vi "INIT TEMP.vi"(8 "error in (no error)":errorcluster, 9 "element":T2 {"Output's Control Loop (1:1)" items=["1"=1, "2"=2]; "Data Source (0:Kelvin)" items=["Kelvin", "Celsius", "Sensor Units"]; "Input (0:A)" items=["A", "B", "C", "D", "D2", "D3", "D4", "D5"]; "Configure Control Parameters (0: Configure)" items=["Configure", "Don't Configure"]; "Serial Configuration"."Flow Control" items=["None", "XON/XOFF", "RTS/CTS", "XON/XOFF & RTS/CTS", "DTR/DSR", "XON/XOFF & DTR/DSR"]; "Serial Configuration"."Stop Bits" items=["1.0"=10, "1.5"=15, "2.0"=20]; "Serial Configuration"."Data Bits" items=["7"=7, "8"=8]; "Serial Configuration"."Parity" items=["None", "Odd", "Even", "Mark", "Space"]; "Serial Configuration"."Baud Rate" items=["300"=300, "600"=600, "1200"=1200, "2400"=2400, "4800"=4800, "9600"=9600, "19200"=19200, "38400"=38400, "57600"=57600]; "Target Temp (K)" format="%.5f"; "Input (0:None)" items=["None", "A", "B", "C", "D", "D2", "D3", "D4", "D5"]; "Mode (0:Off)" items=["Off", "Closed Loop PID", "Zone", "Open Loop"]; "Heater Out Display (1:Current)" items=["Current"=1, "Power"=2]; "Max Current (0:User Specified)" items=["User Specified", "0.707 A", "1.0 A", "1.141 A", "2.0 A"]; "Heater Resistance (1:25 Ohms)" items=["25 Ohms"=1, "50 Ohms"=2]; "Max User Current (2.000)" format="%.3f"; "Gain (P) (50.0)" format="%.1f"; "Reset (I) (20.0)" format="%.1f"; "Rate (D) (0.0 %)" format="%.1f"; "Manual Output (0.00 %)" format="%.2f"; "Range (0:Off)" items=["Off", "Range 1 (On)", "Range 2", "Range 3", "Range 4", "Range 5"]}, 10 "Field and Temp Range":T1={"VISA (Magnet)"="COM4", "Fields(T)"=[], "Temps(K)"=[], "VISA (Temp) "="COM1", "Port number (3364)"=3364}, 11 "Queue in":refnum<queue>) -> (0 "error out":errorcluster, 1 "output cluster":T2={"Range (0:Off)"=0, "Manual Output (0.00 %)"=0.0, "Rate (D) (0.0 %)"=0.0, "Reset (I) (20.0)"=20.0, "Gain (P) (50.0)"=50.0, "Power Up Enable (F: Disable)"=FALSE, "Max User Current (2.000)"=2.0, "Heater Resistance (1:25 Ohms)"=1, "Max Current (0:User Specified)"=0, "Heater Out Display (1:Current)"=1, "Mode (0:Off)"=1, "Input (0:None)"=4, "Target Temp (K)"=5.0, "Serial Configuration"={"Baud Rate"=57600, "Parity"=1, "Data Bits"=7, "Stop Bits"=10, "Flow Control"=0}, "VISA resource name"="", "Configure Control Parameters (0: Configure)"=0, "Enable Setpoint (F:Disable)"=FALSE, "Input (0:A)"=3, "Data Source (0:Kelvin)"=0, "Output's Control Loop (1:1)"=2, "STND DEV Threshold "=0.1, "Mean Tolerance "=0.02, "Current State"=enum."1. INIT TEMP"} {"Output's Control Loop (1:1)" items=["1"=1, "2"=2]; "Data Source (0:Kelvin)" items=["Kelvin", "Celsius", "Sensor Units"]; "Input (0:A)" items=["A", "B", "C", "D", "D2", "D3", "D4", "D5"]; "Configure Control Parameters (0: Configure)" items=["Configure", "Don't Configure"]; "Serial Configuration"."Flow Control" items=["None", "XON/XOFF", "RTS/CTS", "XON/XOFF & RTS/CTS", "DTR/DSR", "XON/XOFF & DTR/DSR"]; "Serial Configuration"."Stop Bits" items=["1.0"=10, "1.5"=15, "2.0"=20]; "Serial Configuration"."Data Bits" items=["7"=7, "8"=8]; "Serial Configuration"."Parity" items=["None", "Odd", "Even", "Mark", "Space"]; "Serial Configuration"."Baud Rate" items=["300"=300, "600"=600, "1200"=1200, "2400"=2400, "4800"=4800, "9600"=9600, "19200"=19200, "38400"=38400, "57600"=57600]; "Target Temp (K)" format="%.5f"; "Input (0:None)" items=["None", "A", "B", "C", "D", "D2", "D3", "D4", "D5"]; "Mode (0:Off)" items=["Off", "Closed Loop PID", "Zone", "Open Loop"]; "Heater Out Display (1:Current)" items=["Current"=1, "Power"=2]; "Max Current (0:User Specified)" items=["User Specified", "0.707 A", "1.0 A", "1.141 A", "2.0 A"]; "Heater Resistance (1:25 Ohms)" items=["25 Ohms"=1, "50 Ohms"=2]; "Max User Current (2.000)" format="%.3f"; "Gain (P) (50.0)" format="%.1f"; "Reset (I) (20.0)" format="%.1f"; "Rate (D) (0.0 %)" format="%.1f"; "Manual Output (0.00 %)" format="%.2f"; "Range (0:Off)" items=["Off", "Range 1 (On)", "Range 2", "Range 3", "Range 4", "Range 5"]}, 2 "VISA resource name out":refnum<visa-resource-name>, 3 "Queue out":refnum<queue>)   [LabVIEW 2025]
uses:
  Downloads/OneDrive_2025-09-03/Instrument Controls/Temp Cntrl.ctl
  <instrlib>/Lake Shore 350/Lake Shore 350.lvlib
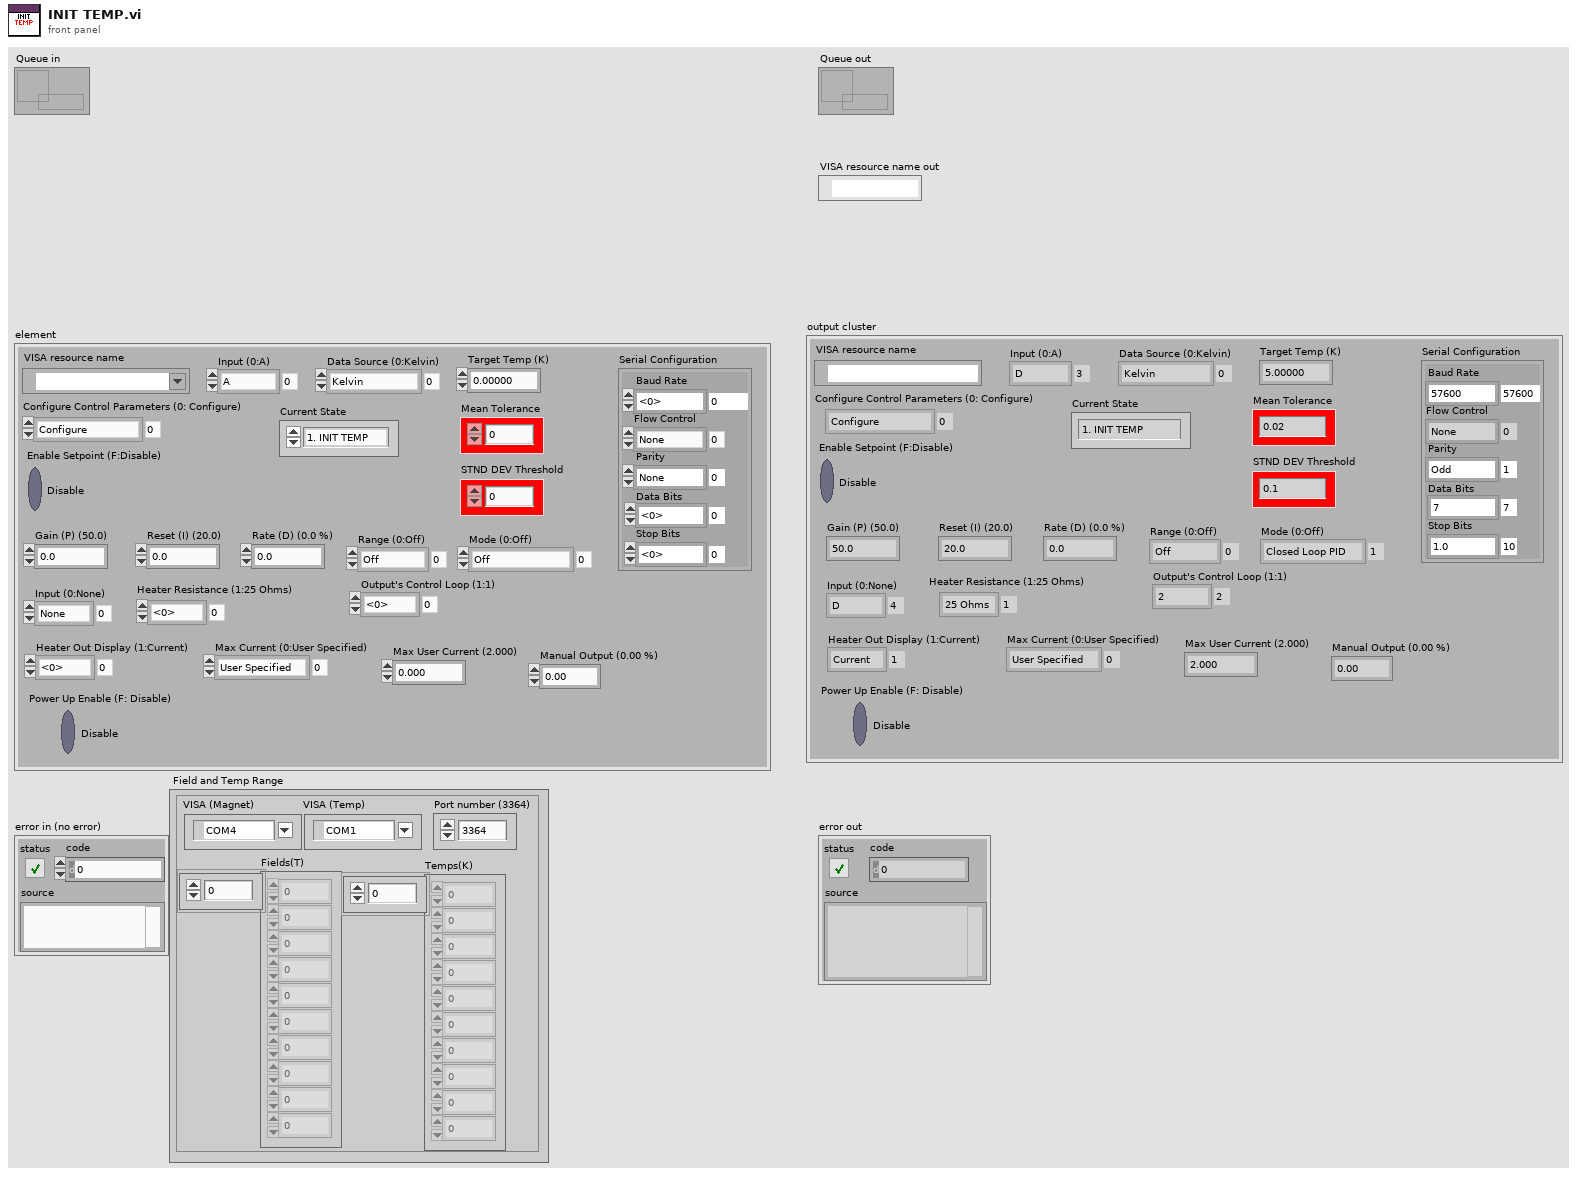
[diagram p1: front panel]
types:
  T1 = cluster{"VISA (Magnet)":refnum<visa-resource-name>, "Fields(T)":dbl[], "Temps(K)":dbl[], "VISA (Temp) ":refnum<visa-resource-name>, "Port number (3364)":u32}
  T2 = typedef "Temp Cntrl.ctl" = cluster{"Range (0:Off)":u16, "Manual Output (0.00 %)":dbl, "Rate (D) (0.0 %)":dbl, "Reset (I) (20.0)":dbl, "Gain (P) (50.0)":dbl, "Power Up Enable (F: Disable)":bool, "Max User Current (2.000)":dbl, "Heater Resistance (1:25 Ohms)":u16, "Max Current (0:User Specified)":u16, "Heater Out Display (1:Current)":u16, "Mode (0:Off)":u16, "Input (0:None)":u16, "Target Temp (K)":dbl, "Serial Configuration":cluster{"Baud Rate":u32, "Parity":u16, "Data Bits":u16, "Stop Bits":u16, "Flow Control":u16}, "VISA resource name":refnum<visa-resource-name>, "Configure Control Parameters (0: Configure)":u16, "Enable Setpoint (F:Disable)":bool, "Input (0:A)":u16, "Data Source (0:Kelvin)":u16, "Output's Control Loop (1:1)":u16, "STND DEV Threshold ":dbl, "Mean Tolerance ":dbl, "Current State":enum16{"1. INIT TEMP", "2. TC ON", "3. POLL_TEMPS", "4. TEMP_STAB", "5. TC IDLE", "6. APPLY NEXT TEMP", "7. TC OFF (Reset)"}}
  T3 = enum16{"1. INIT TEMP", "2. TC ON", "3. POLL_TEMPS", "4. TEMP_STAB", "5. TC IDLE", "6. APPLY NEXT TEMP", "7. TC OFF (Reset)"}
  T4 = cluster{"Baud Rate":u32, "Parity":u16, "Data Bits":u16, "Stop Bits":u16, "Flow Control":u16}
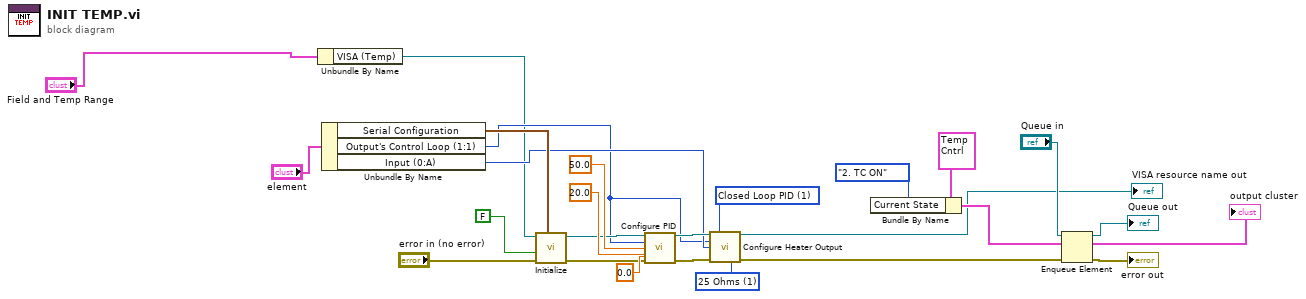
[diagram p0: block diagram]
diagram:
  w7 = u16 1 items=["25 Ohms"=1, "50 Ohms"=2] ("Heater Resistance (1:25 Ohms)")
  w8 = u16 1 items=["Off", "Closed Loop PID", "Zone", "Open Loop"] ("Mode (0:Off)")
  n1 = Unbundle By Name("Field and Temp Range") -> ("VISA (Temp)"=w2:refnum<visa-resource-name>)
  n2 = Unbundle By Name("element") -> ("Serial Configuration"=w17:T4, "Output's Control Loop (1:1)"=w6:u16, "Input (0:A)"=w9:u16)
  n3 = call <instrlib>:"Initialize.vi"("Serial Configuration"=w17, "error in (no error)"="error in (no error)", "Reset (True)"=FALSE, "VISA resource name"=w2) -> ("error out"=w15:errorcluster, "VISA resource name out"=w14:refnum<visa-resource-name>)  [unwired: 6 in]
  n4 = call <instrlib>:"Configure PID.vi"("VISA resource name"=w14, "Output's Control Loop (1:1)"=w6, "Gain (P) (50.0)"=50.0, "Reset (I) (20.0)"=20.0, "error in (no error)"=w15, "Rate (D) (0.0 %)"=0.0) -> ("VISA resource name out"=w11:refnum<visa-resource-name>, "error out"=w10:errorcluster)  [unwired: 8 in]
  n5 = call <instrlib>:"Configure Heater Output.vi"("VISA resource name"=w11, "Mode (0:Off)"=w8, "Heater Output (1:1)"=w6, "Input (0:None)"=w9, "error in (no error)"=w10, "Heater Resistance (1:25 Ohms)"=w7) -> ("VISA resource name out"=→"VISA resource name out":refnum<visa-resource-name>, "error out"=w5:errorcluster)  [unwired: 8 in]
  n6 = Bundle By Name(cluster=T2 {"Range (0:Off)"=0, "Manual Output (0.00 %)"=0.0, "Rate (D) (0.0 %)"=0.0, "Reset (I) (20.0)"=20.0, "Gain (P) (50.0)"=50.0, "Power Up Enable (F: Disable)"=FALSE, "Max User Current (2.000)"=2.0, "Heater Resistance (1:25 Ohms)"=1, "Max Current (0:User Specified)"=0, "Heater Out Display (1:Current)"=1, "Mode (0:Off)"=1, "Input (0:None)"=4, "Target Temp (K)"=5.0, "Serial Configuration"={"Baud Rate"=57600, "Parity"=1, "Data Bits"=7, "Stop Bits"=10, "Flow Control"=0}, "VISA resource name"="", "Configure Control Parameters (0: Configure)"=0, "Enable Setpoint (F:Disable)"=FALSE, "Input (0:A)"=3, "Data Source (0:Kelvin)"=0, "Output's Control Loop (1:1)"=2, "STND DEV Threshold "=0.1, "Mean Tolerance "=0.02, "Current State"=enum."1. INIT TEMP"} ("element"), "Current State"=T3."2. TC ON") -> (w23:T2)
  "output cluster" <- w23
  n7 = Enqueue Element(queue="Queue in", element=w23, error in (no error)=w5) -> (queue out=→"Queue out":refnum<queue>, error out=→"error out":errorcluster)  [unwired: 1 in, 1 out]
